vi "ConnTemplateTest.vi"(0 "Shape":refnum<class "Connection-t'Function Generator.lvlib-Shape.ctl'.lvclass">, 1 "Sample Rate":dbl, 2 "Sample Count":dbl, 5 "Frequency":refnum<class "Connection-dbl.lvclass">, 7 "Amplitude":refnum<class "Connection-dbl.lvclass">, 9 "Phase":refnum<class "Connection-dbl.lvclass">, 11 "Offset":refnum<class "Connection-dbl.lvclass">) -> (4 "Out":refnum<class "Connection-c(dbl,dbl,a[.](cdb)).lvclass">)   [LabVIEW 2020]
uses:
  <extravilib>/Connections/Connection-t'Function Generator.lvlib-Shape.ctl'.lvclass
  <extravilib>/Connections/Connection-dbl.lvclass
  <extravilib>/Connections/Connection-c(dbl,dbl,a[.](cdb)).lvclass
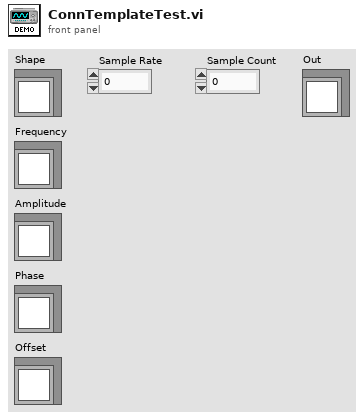
[diagram p1: front panel]
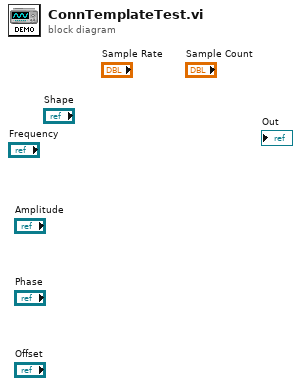
[diagram p0: block diagram]
diagram:
